vi "U3 Read CalMem.vi"() -> ()   [LabVIEW 2021]
panel:
  out "Array Read":dbl[](array[numeric])
  out "Error Message":string
  out "error out":errorcluster
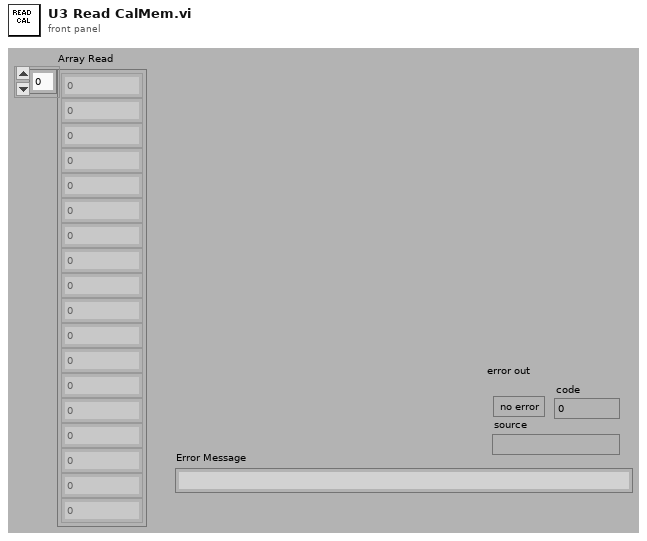
[diagram p1: front panel]
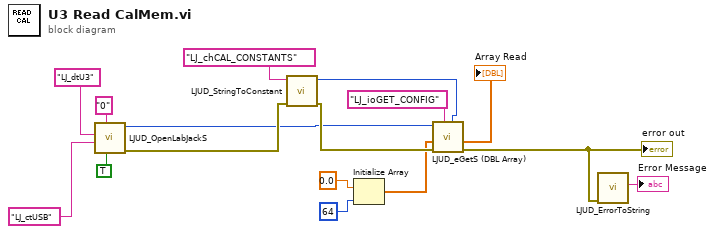
[diagram p0: block diagram]
diagram:
  n1 = call "LJUD_OpenLabJackS.vi"("FirstFound"=TRUE, "Address"="0", "ConnectionType"="LJ_ctUSB", "DeviceType"="LJ_dtU3") -> ("error out"=w4:errorcluster, "Handle"=w3:i32)  [unwired: 5 in, 1 out]
  n2 = call "LJUD_StringToConstant.vi"("error in"=w4, "String"="LJ_chCAL_CONSTANTS") -> ("error out"=w6:errorcluster, "Constant Number"=w7:i32)  [unwired: 8 in]
  n3 = Initialize Array(0.0 ("dimension size"), 64 ("# Elements")) -> (w5:dbl[])
  n4 = call "LJUD_eGetS (DBL Array).vi"("Channel"=w7, "IOType"="LJ_ioGET_CONFIG", "error in"=w6, "DBL Array Write"=w5, "Handle In"=w3) -> ("error out"=w14:errorcluster, "DBL Array Read"=→"Array Read":dbl[])  [unwired: 3 in, 2 out]
  "error out" <- w14
  n5 = call "LJUD_ErrorToString.vi"("error in"=w14) -> ("String"=→"Error Message":string)  [unwired: 10 in]
